vi "rsscope_core_global.vi"() -> ()   [LabVIEW 2014] (continued)
"Descriptive Name"="Advanced Jitter Gating Coupled Zoom Diagram", "Data Type"=6, "Command"="ADVJ{AdvJitterMeas}:SIGN:GATE:ZDI", "Access"=2, "Range Table"="", "Read Callback"="", "Write Callback"="", "Supported Models"="", "Instrument Options"="K133|K134", "Flags"=0, "Help"="Sets the zoom the gate is coupled to, if RSSCOPE_ATTR_ADVANCED_JITTER_GATING_COUPLING_MODE is set to ZOOM.\n\nAvailable Repeated Capabilities:\nAdvJitterMeas: JA1, JA2\r\n\nRemote-control command(s):\nADVJitter<m>:SIGNal:GATE:ZDIagram"}, {"Level"=5, "Class Only"=FALSE, "Identifier"="RSSCOPE_ATTR_ADVANCED_JITTER_GATING_MODE", "Descriptive Name"="Advanced Jitter Gating Mode", "Data Type"=0, "Command"="ADVJ{AdvJitterMeas}:SIGN:GATE:RANG:MODE", "Access"=2, "Range Table"="rsscope_rngAbsRel", "Read Callback"="", "Write Callback"="", "Supported Models"="", "Instrument Options"="K133|K134", "Flags"=0, "Help"="Selects if the gate area is defined in relative values (percent) or absolute.\n\nAvailable Repeated Capabilities:\nAdvJitterMeas: JA1, JA2\r\n\nRemote-control command(s):\nADVJitter<m>:SIGNal:GATE:RANGe:MODE"}, {"Level"=5, "Class Only"=FALSE, "Identifier"="RSSCOPE_ATTR_ADVANCED_JITTER_GATING_ABSOLUTE_START", "Descriptive Name"="Advanced Jitter Gating Absolute Start", "Data Type"=1, "Command"="ADVJ{AdvJitterMeas}:SIGN:GATE:RANG:ABS:STAR", "Access"=2, "Range Table"="RsScope_rngAdvancedJitterGatingRange", "Read Callback"="", "Write Callback"="", "Supported Models"="", "Instrument Options"="K133|K134", "Flags"=0, "Help"="Sets the start time of the gate area in percent, if RSSCOPE_ATTR_ADVANCED_JITTER_GATING_MODE is set to ABS.\n\nAvailable Repeated Capabilities:\nAdvJitterMeas: JA1, JA2\r\n\nRemote-control command(s):\nADVJitter<m>:SIGNal:GATE:RANGe:ABSolute:STARt"}, {"Level"=5, "Class Only"=FALSE, "Identifier"="RSSCOPE_ATTR_ADVANCED_JITTER_GATING_ABSOLUTE_STOP", "Descriptive Name"="Advanced Jitter Gating Absolute Stop", "Data Type"=1, "Command"="ADVJ{AdvJitterMeas}:SIGN:GATE:RANG:ABS:STOP", "Access"=2, "Range Table"="RsScope_rngAdvancedJitterGatingRange", "Read Callback"="", "Write Callback"="", "Supported Models"="", "Instrument Options"="K133|K134", "Flags"=0, "Help"="Sets the stop time of the gate area in percent, if RSSCOPE_ATTR_ADVANCED_JITTER_GATING_MODE is set to ABS.\n\nAvailable Repeated Capabilities:\nAdvJitterMeas: JA1, JA2\r\n\nRemote-control command(s):\nADVJitter<m>:SIGNal:GATE:RANGe:ABSolute:STOP"}, {"Level"=5, "Class Only"=FALSE, "Identifier"="RSSCOPE_ATTR_ADVANCED_JITTER_GATING_RELATIVE_START", "Descriptive Name"="Advanced Jitter Gating Relative Start", "Data Type"=1, "Command"="ADVJ{AdvJitterMeas}:SIGN:GATE:RANG:REL:STAR", "Access"=2, "Range Table"="RsScope_rngPercent", "Read Callback"="", "Write Callback"="", "Supported Models"="", "Instrument Options"="K133|K134", "Flags"=0, "Help"="Sets the relative start of the gate area in percent, if RSSCOPE_ATTR_ADVANCED_JITTER_GATING_MODE is set to REL.\n\nAvailable Repeated Capabilities:\nAdvJitterMeas: JA1, JA2\r\n\nRemote-control command(s):\nADVJitter<m>:SIGNal:GATE:RANGe:RELative:STARt"}, {"Level"=5, "Class Only"=FALSE, "Identifier"="RSSCOPE_ATTR_ADVANCED_JITTER_GATING_RELATIVE_STOP", "Descriptive Name"="Advanced Jitter Gating Relative Stop", "Data Type"=1, "Command"="ADVJ{AdvJitterMeas}:SIGN:GATE:RANG:REL:STOP", "Access"=2, "Range Table"="RsScope_rngPercent", "Read Callback"="", "Write Callback"="", "Supported Models"="", "Instrument Options"="K133|K134", "Flags"=0, "Help"="Sets the relative stop of the gate area in percent, if RSSCOPE_ATTR_ADVANCED_JITTER_GATING_MODE is set to REL.\n\nAvailable Repeated Capabilities:\nAdvJitterMeas: JA1, JA2\r\n\nRemote-control command(s):\nADVJitter<m>:SIGNal:GATE:RANGe:RELative:STOP"}, {"Level"=4, "Class Only"=TRUE, "Identifier"="", "Descriptive Name"="Decomposition", "Data Type"=0, "Command"="", "Access"=0, "Range Table"="", "Read Callback"="", "Write Callback"="", "Supported Models"="", "Instrument Options"="", "Flags"=0, "Help"="This class contains attributes and methods to set the step response of the system and select the jitter components measurements that you want to perform in the advanced jitter measurement subsystem (option K133)"}, {"Level"=5, "Class Only"=FALSE, "Identifier"="RSSCOPE_ATTR_ADVANCED_JITTER_DECOMPOSITION_STEP_RESPONSE_LENGTH", "Descriptive Name"="Advanced Jitter Decomposition Step Response Length", "Data Type"=1, "Command"="ADVJ{AdvJitterMeas}:DCOM:RESP", "Access"=2, "Range Table"="RsScope_rngAdvancedJitterStepResponse", "Read Callback"="", "Write Callback"="", "Supported Models"="", "Instrument Options"="K133|K134", "Flags"=0, "Help"="Set the  step response length in unit intervals.\n\nAvailable Repeated Capabilities:\nAdvJitterMeas: JA1, JA2\r\n\nRemote-control command(s):\nADVJitter<m>:DCOMposition:RESPlength"}, {"Level"=5, "Class Only"=FALSE, "Identifier"="RSSCOPE_ATTR_ADVANCED_JITTER_DECOMPOSITION_ESTIMATE_STEP_RESPONSE", "Descriptive Name"="Advanced Jitter Decomposition Estimate Step Response", "Data Type"=4, "Command"="ADVJ{AdvJitterMeas}:DCOM:RLES", "Access"=1, "Range Table"="", "Read Callback"="", "Write Callback"="", "Supported Models"="", "Instrument Options"="K133|K134", "Flags"=1, "Help"="Estimates the maximum of the reasonable step response length depending on the analyzed signal that guarantees the calculation of the step responses. Tor this, however, a smaller value is also possible, which can be set user-defined with RSSCOPE_ATTR_ADVANCED_JITTER_DECOMPOSITION_STEP_RESPONSE_LENGTH. The user-defined value is overwritten if the estimated maximum is less than the value set by the user.\n\nAvailable Repeated Capabilities:\nAdvJitterMeas: JA1, JA2\r\n\nRemote-control command(s):\nADVJitter<m>:DCOMposition:RLEStimate"}, {"Level"=5, "Class Only"=FALSE, "Identifier"="RSSCOPE_ATTR_ADVANCED_JITTER_DECOMPOSITION_STEP_RESPONSE_ESTIMATED_MAX", "Descriptive Name"="Advanced Jitter Decomposition Step Response Estimated Max", "Data Type"=1, "Command"="ADVJ{AdvJitterMeas}:DCOM:MRES?", "Access"=0, "Range Table"="RsScope_rngAdvancedJitterStepResponse", "Read Callback"="", "Write Callback"="", "Supported Models"="", "Instrument Options"="K133|K134", "Flags"=0, "Help"="Queries the estimated maximum step length response.\n\nAvailable Repeated Capabilities:\nAdvJitterMeas: JA1, JA2\r\n\nRemote-control command(s):\nADVJitter<m>:DCOMposition:MRESplength?"}, {"Level"=5, "Class Only"=FALSE, "Identifier"="RSSCOPE_ATTR_ADVANCED_JITTER_DECOMPOSITION_STEP_POSITION", "Descriptive Name"="Advanced Jitter Decomposition Step Position", "Data Type"=0, "Command"="ADVJ{AdvJitterMeas}:DCOM:POSS", "Access"=2, "Range Table"="rsscope_rngPct", "Read Callback"="", "Write Callback"="", "Supported Models"="", "Instrument Options"="K133|K134", "Flags"=0, "Help"="Sets the steps position. It defines what percentage of the unit lengths are displayed before the step response.\n\nFor example, if the Length is set to 20 UI and the Step position is set to 75%, the step response diagram displays 15 UI before the step response and 5 UI after that.\n\nAvailable Repeated Capabilities:\nAdvJitterMeas: JA1, JA2\r\n\nRemote-control command(s):\nADVJitter<m>:DCOMposition:POSStep"}, {"Level"=5, "Class Only"=FALSE, "Identifier"="RSSCOPE_ATTR_ADVANCED_JITTER_DECOMPOSITION_TARGET_BER_EXPONENT", "Descriptive Name"="Advanced Jitter Decomposition Target BER Exponent", "Data Type"=0, "Command"="ADVJ{AdvJitterMeas}:DCOM:TARB", "Access"=2, "Range Table"="RsScope_rngAdvancedJitterTargetBERExponent", "Read Callback"="", "Write Callback"="", "Supported Models"="", "Instrument Options"="K133|K134", "Flags"=0, "Help"="Sets the target bit error rate for total jitter at BER components. This value is the exponent n where BER = 10^-n.\n\nAvailable Repeated Capabilities:\nAdvJitterMeas: JA1, JA2\r\n\nRemote-control command(s):\nADVJitter<m>:DCOMposition:TARBer"}, {"Level"=5, "Class Only"=FALSE, "Identifier"="RSSCOPE_ATTR_ADVANCED_JITTER_DECOMPOSITION_DISPLAY_INTERLEAVED", "Descriptive Name"="Advanced Jitter Decomposition Display Interleaved", "Data Type"=3, "Command"="ADVJ{AdvJitterMeas}:DCOM:JINT", "Access"=2, "Range Table"="", "Read Callback"="", "Write Callback"="", "Supported Models"="", "Instrument Options"="K133|K134", "Flags"=0, "Help"="Displays interleaved histogram values.\n\nAvailable Repeated Capabilities:\nAdvJitterMeas: JA1, JA2\r\n\nRemote-control command(s):\nADVJitter<m>:DCOMposition:JINTerleaved"}, {"Level"=5, "Class Only"=FALSE, "Identifier"="RSSCOPE_ATTR_ADVANCED_JITTER_DECOMPOSITION_DISPLAY_PERIODIC_JITTER_LABELS", "Descriptive Name"="Advanced Jitter Decomposition Display Periodic Jitter Labels", "Data Type"=3, "Command"="ADVJ{AdvJitterMeas}:DCOM:SPJL", "Access"=2, "Range Table"="", "Read Callback"="", "Write Callback"="", "Supported Models"="", "Instrument Options"="K133|K134", "Flags"=0, "Help"="Enables the display of the periodic jitter components labels.\n\nAvailable Repeated Capabilities:\nAdvJitterMeas: JA1, JA2\r\n\nRemote-control command(s):\nADVJitter<m>:DCOMposition:SPJLabels"}, {"Level"=5, "Class Only"=FALSE, "Identifier"="RSSCOPE_ATTR_ADVANCED_JITTER_DECOMPOSITION_DISPLAY_PERIODIC_NOISE_LABELS", "Descriptive Name"="Advanced Jitter Decomposition Display Periodic Noise Labels", "Data Type"=3, "Command"="ADVJ{AdvJitterMeas}:DCOM:SPNL", "Access"=2, "Range Table"="", "Read Callback"="", "Write Callback"="", "Supported Models"="", "Instrument Options"="K133|K134", "Flags"=0, "Help"="Enables the display of the periodic noise components labels.\n\nAvailable Repeated Capabilities:\nAdvJitterMeas: JA1, JA2\r\n\nRemote-control command(s):\nADVJitter<m>:DCOMposition:SPNLabels"}, {"Level"=5, "Class Only"=TRUE, "Identifier"="", "Descriptive Name"="Components", "Data Type"=0, "Command"="", "Access"=0, "Range Table"="", "Read Callback"="", "Write Callback"="", "Supported Models"="", "Instrument Options"="", "Flags"=0, "Help"="This class contains methods that enable and configure jitter decomposition components in the advanced jitter measurement subsystem (option K133)"}, {"Level"=6, "Class Only"=FALSE, "Identifier"="RSSCOPE_ATTR_ADVANCED_JITTER_DECOMPOSITION_SELECT_ALL_BASIC_JITTER_COMPONENTS", "Descriptive Name"="Advanced Jitter Decomposition Select All Basic Jitter Components", "Data Type"=4, "Command"="ADVJ{AdvJitterMeas}:DCOM:SELB", "Access"=1, "Range Table"="", "Read Callback"="", "Write Callback"="", "Supported Models"="", "Instrument Options"="K133|K134", "Flags"=0, "Help"="Selects all basic jitter components.\n\nAvailable Repeated Capabilities:\nAdvJitterMeas: JA1, JA2\r\n\nRemote-control command(s):\nADVJitter<m>:DCOMposition:SELBasicmeas"}, {"Level"=6, "Class Only"=FALSE, "Identifier"="RSSCOPE_ATTR_ADVANCED_JITTER_DECOMPOSITION_SELECT_ALL_JITTER_COMPONENTS", "Descriptive Name"="Advanced Jitter Decomposition Select All Jitter Components", "Data Type"=4, "Command"="ADVJ{AdvJitterMeas}:DCOM:SELJ", "Access"=1, "Range Table"="", "Read Callback"="", "Write Callback"="", "Supported Models"="", "Instrument Options"="K133|K134", "Flags"=0, "Help"="Selects all jitter components.\n\nAvailable Repeated Capabilities:\nAdvJitterMeas: JA1, JA2\r\n\nRemote-control command(s):\nADVJitter<m>:DCOMposition:SELJitcomp"}, {"Level"=6, "Class Only"=FALSE, "Identifier"="RSSCOPE_ATTR_ADVANCED_JITTER_DECOMPOSITION_CLEAR_SELECTED_BASIC_JITTER_COMPONENTS", "Descriptive Name"="Advanced Jitter Decomposition Clear Selected Basic Jitter Components", "Data Type"=4, "Command"="ADVJ{AdvJitterMeas}:DCOM:CLEB", "Access"=1, "Range Table"="", "Read Callback"="", "Write Callback"="", "Supported Models"="", "Instrument Options"="K133|K134", "Flags"=0, "Help"="Clears all selected basic jitter components.\n\nAvailable Repeated Capabilities:\nAdvJitterMeas: JA1, JA2\r\n\nRemote-control command(s):\nADVJitter<m>:DCOMposition:CLEBasicmeas"}, {"Level"=6, "Class Only"=FALSE, "Identifier"="RSSCOPE_ATTR_ADVANCED_JITTER_DECOMPOSITION_CLEAR_SELECTED_JITTER_COMPONENTS", "Descriptive Name"="Advanced Jitter Decomposition Clear Selected Jitter Components", "Data Type"=4, "Command"="ADVJ{AdvJitterMeas}:DCOM:CLEJ", "Access"=1, "Range Table"="", "Read Callback"="", "Write Callback"="", "Supported Models"="", "Instrument Options"="K133|K134", "Flags"=0, "Help"="Clears all selected jitter components.\n\nAvailable Repeated Capabilities:\nAdvJitterMeas: JA1, JA2\r\n\nRemote-control command(s):\nADVJitter<m>:DCOMposition:CLEJitcomp"}, {"Level"=6, "Class Only"=FALSE, "Identifier"="RSSCOPE_ATTR_ADVANCED_JITTER_DECOMPOSITION_COMPONENT_ENABLED", "Descriptive Name"="Advanced Jitter Decomposition Component Enabled", "Data Type"=3, "Command"="ADVJ{AdvJitterMeas}:DCOM:COMP{AdvJitterComponent}:ENAB", "Access"=2, "Range Table"="", "Read Callback"="", "Write Callback"="", "Supported Models"="", "Instrument Options"="K133|K134", "Flags"=0, "Help"="Enables the measurement for the specified jitter component.\n\nAvailable Repeated Capabilities:\nAdvJitterMeas: JA1, JA2\r\nAdvJitterComponent: f_symb, T_symb, EC, TJ_BER, RJ, DDirac, TJ, DJ, DDJ, DCD, PJ, ISI\r\n\nRemote-control command(s):\nADVJitter<m>:DCOMposition:COMPonents<n>:ENABle"}, {"Level"=6, "Class Only"=FALSE, "Identifier"="RSSCOPE_ATTR_ADVANCED_JITTER_DECOMPOSITION_SELECT_ALL_NOISE_COMPONENTS", "Descriptive Name"="Advanced Jitter Decomposition Select All Noise Components", "Data Type"=4, "Command"="ADVJ{AdvJitterMeas}:DCOM:SELN", "Access"=1, "Range Table"="", "Read Callback"="", "Write Callback"="", "Supported Models"="", "Instrument Options"="K133|K134", "Flags"=0, "Help"="Selects all noise components.\n\nAvailable Repeated Capabilities:\nAdvJitterMeas: JA1, JA2\r\n\nRemote-control command(s):\nADVJitter<m>:DCOMposition:SELNoisecomp"}, {"Level"=6, "Class Only"=FALSE, "Identifier"="RSSCOPE_ATTR_ADVANCED_JITTER_DECOMPOSITION_CLEAR_SELECTED_NOISE_COMPONENTS", "Descriptive Name"="Advanced Jitter Decomposition Clear Selected Noise Components", "Data Type"=4, "Command"="ADVJ{AdvJitterMeas}:DCOM:CLEN", "Access"=1, "Range Table"="", "Read Callback"="", "Write Callback"="", "Supported Models"="", "Instrument Options"="K133|K134", "Flags"=0, "Help"="Clears all selected noise components.\n\nAvailable Repeated Capabilities:\nAdvJitterMeas: JA1, JA2\r\n\nRemote-control command(s):\nADVJitter<m>:DCOMposition:CLENoisecomp"}, {"Level"=6, "Class Only"=FALSE, "Identifier"="RSSCOPE_ATTR_ADVANCED_JITTER_DECOMPOSITION_PERIODIC_COMPONENTS_ENABLED", "Descriptive Name"="Advanced Jitter Decomposition Periodic Components Enabled", "Data Type"=3, "Command"="ADVJ{AdvJitterMeas}:DCOM:ENP", "Access"=2, "Range Table"="", "Read Callback"="", "Write Callback"="", "Supported Models"="", "Instrument Options"="K133|K134", "Flags"=0, "Help"="Enables the display of the periodic jitter components table.\n\nAvailable Repeated Capabilities:\nAdvJitterMeas: JA1, JA2\r\n\nRemote-control command(s):\nADVJitter<m>:DCOMposition:ENP"}, {"Level"=6, "Class Only"=FALSE, "Identifier"="RSSCOPE_ATTR_ADVANCED_JITTER_DECOMPOSITION_MAX_PERIODIC_VERTICAL_COMPONENTS", "Descriptive Name"="Advanced Jitter Decomposition Max Periodic Vertical Components", "Data Type"=0, "Command"="ADVJ{AdvJitterMeas}:DCOM:NVER", "Access"=2, "Range Table"="RsScope_rngAdvancedJitterPeriodicComponents", "Read Callback"="", "Write Callback"="", "Supported Models"="", "Instrument Options"="K133|K134", "Flags"=0, "Help"="Sets the maximum number of periodic components in the vertical direction that are considered for the measurement. If the actual number of periodic components is higher than the set value, they are considered for the random jitter component.\n\nAvailable Repeated Capabilities:\nAdvJitterMeas: JA1, JA2\r\n\nRemote-control command(s):\nADVJitter<m>:DCOMposition:NVERtical"}, {"Level"=6, "Class Only"=FALSE, "Identifier"="RSSCOPE_ATTR_ADVANCED_JITTER_DECOMPOSITION_MAX_PERIODIC_HORIZONTAL_COMPONENTS", "Descriptive Name"="Advanced Jitter Decomposition Max Periodic Horizontal Components", "Data Type"=0, "Command"="ADVJ{AdvJitterMeas}:DCOM:NHOR", "Access"=2, "Range Table"="RsScope_rngAdvancedJitterPeriodicComponents", "Read Callback"="", "Write Callback"="", "Supported Models"="", "Instrument Options"="K133|K134", "Flags"=0, "Help"="Sets the maximum number of periodic components in the horizontal direction that are considered for the measurement. If the actual number of periodic components is higher than the set value, they are considered for the random jitter component.\n\nAvailable Repeated Capabilities:\nAdvJitterMeas: JA1, JA2\r\n\nRemote-control command(s):\nADVJitter<m>:DCOMposition:NHORizontal"}, {"Level"=6, "Class Only"=FALSE, "Identifier"="RSSCOPE_ATTR_ADVANCED_JITTER_DECOMPOSITION_OTHER_BOUNDED_UNCORRELATED_ENABLED", "Descriptive Name"="Advanced Jitter Decomposition Other Bounded Uncorrelated Enabled", "Data Type"=3, "Command"="ADVJ{AdvJitterMeas}:DCOM:ENOB", "Access"=2, "Range Table"="", "Read Callback"="", "Write Callback"="", "Supported Models"="", "Instrument Options"="K133|K134", "Flags"=0, "Help"="If enabled, allows the selection of the (other) bounded uncorrelated jitter/noise: (O)BUJ, (O)BUJ(d -d) , RJ, (O)BUN, (O)BUN(d -d) , RN.\n\nThe other bounded uncorrelated jitter/noise includes the periodic jitter/noise components. It is displayed, if Periodic is enabled. Otherwise the bounded uncorrelated jitter/noise is displayed.\n\nAvailable Repeated Capabilities:\nAdvJitterMeas: JA1, JA2\r\n\nRemote-control command(s):\nADVJitter<m>:DCOMposition:ENOBu"}, {"Level"=6, "Class Only"=FALSE, "Identifier"="RSSCOPE_ATTR_ADVANCED_JITTER_DECOMPOSITION_PERIODIC_JITTER_TABLE_ENABLED", "Descriptive Name"="Advanced Jitter Decomposition Periodic Jitter Table Enabled", "Data Type"=3, "Command"="ADVJ{AdvJitterMeas}:DCOM:SPJT", "Access"=2, "Range Table"="", "Read Callback"="", "Write Callback"="", "Supported Models"="", "Instrument Options"="K133|K134", "Flags"=0, "Help"="Enables the display of the periodic jitter components table.\n\nAvailable Repeated Capabilities:\nAdvJitterMeas: JA1, JA2\r\n\nRemote-control command(s):\nADVJitter<m>:DCOMposition:SPJTable"}, {"Level"=4, "Class Only"=TRUE, "Identifier"="", "Descriptive Name"="Results", "Data Type"=0, "Command"="", "Access"=0, "Range Table"="", "Read Callback"="", "Write Callback"="", "Supported Models"="", "Instrument Options"="", "Flags"=0, "Help"="This class provides access to your measurement results in the advanced jitter measurement subsystem (option K133)"}, {"Level"=5, "Class Only"=FALSE, "Identifier"="RSSCOPE_ATTR_ADVANCED_JITTER_RESULTS_ENABLED", "Descriptive Name"="Advanced Jitter Results Enabled", "Data Type"=3, "Command"="ADVJ{AdvJitterMeas}:RES:ENAB", "Access"=2, "Range Table"="", "Read Callback"="", "Write Callback"="", "Supported Models"="", "Instrument Options"="K133|K134", "Flags"=0, "Help"="Enables the advanced jitter analysis. It displays all enabled diagrams and displays a table with the results for the component measurements.\n\nAvailable Repeated Capabilities:\nAdvJitterMeas: JA1, JA2\r\n\nRemote-control command(s):\nADVJitter<m>:RESult:ENABle"}, {"Level"=5, "Class Only"=FALSE, "Identifier"="RSSCOPE_ATTR_ADVANCED_JITTER_RESULTS_STATISTICS_ENABLED", "Descriptive Name"="Advanced Jitter Results Statistics Enabled", "Data Type"=3, "Command"="ADVJ{AdvJitterMeas}:RES:STAT", "Access"=2, "Range Table"="", "Read Callback"="", "Write Callback"="", "Supported Models"="", "Instrument Options"="K133|K134", "Flags"=0, "Help"="Enables statistics measurements for the advanced jitter analysis.\n\nAvailable Repeated Capabilities:\nAdvJitterMeas: JA1, JA2\r\n\nRemote-control command(s):\nADVJitter<m>:RESult:STATistics"}, {"Level"=5, "Class Only"=FALSE, "Identifier"="RSSCOPE_ATTR_ADVANCED_JITTER_RESULTS_STEP_RESPONSE_DIAGRAM_ENABLED", "Descriptive Name"="Advanced Jitter Results Step Response Diagram Enabled", "Data Type"=3, "Command"="ADVJ{AdvJitterMeas}:RES:STEP", "Access"=2, "Range Table"="", "Read Callback"="", "Write Callback"="", "Supported Models"="", "Instrument Options"="K133|K134", "Flags"=0, "Help"="Enables a step response diagram for the advanced jitter measurements.\n\nAvailable Repeated Capabilities:\nAdvJitterMeas: JA1, JA2\r\n\nRemote-control command(s):\nADVJitter<m>:RESult:STEPresponse"}, {"Level"=5, "Class Only"=FALSE, "Identifier"="RSSCOPE_ATTR_ADVANCED_JITTER_RESULTS_BATHTUB_PLOT_ENABLED", "Descriptive Name"="Advanced Jitter Results Bathtub Plot Enabled", "Data Type"=3, "Command"="ADVJ{AdvJitterMeas}:RES:BATH", "Access"=2, "Range Table"="", "Read Callback"="", "Write Callback"="", "Supported Models"="", "Instrument Options"="K133|K134", "Flags"=0, "Help"="Enables a bathtub plot for the advanced jitter measurements.\n\nAvailable Repeated Capabilities:\nAdvJitterMeas: JA1, JA2\r\n\nRemote-control command(s):\nADVJitter<m>:RESult:BATHtub"}, {"Level"=5, "Class Only"=FALSE, "Identifier"="RSSCOPE_ATTR_ADVANCED_JITTER_RESULTS_BATHTUB_PLOT_TYPE", "Descriptive Name"="Advanced Jitter Results Bathtub Plot Type", "Data Type"=0, "Command"="ADVJ{AdvJitterMeas}:RES:TYPB", "Access"=2, "Range Table"="RsScope_rngAdvancedJitterResultsBathtubPlotType", "Read Callback"="", "Write Callback"="", "Supported Models"="", "Instrument Options"="K133|K134", "Flags"=0, "Help"="Selects if you want to display the bathtub results versus total jitter (TJ) or data-dependent jitter (DDJ) and random jitter (RJ) components.\n\nAvailable Repeated Capabilities:\nAdvJitterMeas: JA1, JA2\r\n\nRemote-control command(s):\nADVJitter<m>:RESult:TYPBathtub"}, {"Level"=5, "Class Only"=FALSE, "Identifier"="RSSCOPE_ATTR_ADVANCED_JITTER_RESULTS_BATHTUB_PERIODIC_COMPONENTS_ENABLED", "Descriptive Name"="Advanced Jitter Results Bathtub Periodic Components Enabled", "Data Type"=3, "Command"="ADVJ{AdvJitterMeas}:RES:PJ", "Access"=2, "Range Table"="", "Read Callback"="", "Write Callback"="", "Supported Models"="", "Instrument Options"="K133|K134", "Flags"=0, "Help"="If enabled, the periodic jitter components are considered for the jitter bathtub. Requires periodic components to be enabled (RSSCOPE_ATTR_ADVANCED_JITTER_DECOMPOSITION_PERIODIC_COMPONENTS_ENABLED).\n\nAvailable Repeated Capabilities:\nAdvJitterMeas: JA1, JA2\r\n\nRemote-control command(s):\nADVJitter<m>:RESult:PJ"}, {"Level"=5, "Class Only"=FALSE, "Identifier"="RSSCOPE_ATTR_ADVANCED_JITTER_RESULTS_BATHTUB_OBUJ_COMPONENTS_ENABLED", "Descriptive Name"="Advanced Jitter Results Bathtub OBUJ Components Enabled", "Data Type"=3, "Command"="ADVJ{AdvJitterMeas}:RES:OBUJ", "Access"=2, "Range Table"="", "Read Callback"="", "Write Callback"="", "Supported Models"="", "Instrument Options"="K133|K134", "Flags"=0, "Help"="If enabled, the other bounded uncorrelated jitter components are considered for the jitter bathtub. Requires other bounded uncorrelated components to be enabled (RSSCOPE_ATTR_ADVANCED_JITTER_DECOMPOSITION_OTHER_BOUNDED_UNCORRELATED_ENABLED).\n\nAvailable Repeated Capabilities:\nAdvJitterMeas: JA1, JA2\r\n\nRemote-control command(s):\nADVJitter<m>:RESult:OBUJ"}, {"Level"=5, "Class Only"=FALSE, "Identifier"="RSSCOPE_ATTR_ADVANCED_JITTER_RESULTS_NOISE_BATHTUB_PLOT_ENABLED", "Descriptive Name"="Advanced Jitter Results Noise Bathtub Plot Enabled", "Data Type"=3, "Command"="ADVJ{AdvJitterMeas}:RES:NBAT", "Access"=2, "Range Table"="", "Read Callback"="", "Write Callback"="", "Supported Models"="", "Instrument Options"="K133|K134", "Flags"=0, "Help"="Enables a noise bathtub plot, a graph of BER in a log scale versus data-dependent jitter (DDN).\n\nAvailable Repeated Capabilities:\nAdvJitterMeas: JA1, JA2\r\n\nRemote-control command(s):\nADVJitter<m>:RESult:NBAThtub"}, {"Level"=5, "Class Only"=FALSE, "Identifier"="RSSCOPE_ATTR_ADVANCED_JITTER_RESULTS_NOISE_BATHTUB_PERIODIC_COMPONENTS_ENABLED", "Descriptive Name"="Advanced Jitter Results Noise Bathtub Periodic Components Enabled", "Data Type"=3, "Command"="ADVJ{AdvJitterMeas}:RES:PN", "Access"=2, "Range Table"="", "Read Callback"="", "Write Callback"="", "Supported Models"="", "Instrument Options"="K133|K134", "Flags"=0, "Help"="If enabled, the periodic noise components are considered for the noise bathtub. Requires periodic components to be enabled (RSSCOPE_ATTR_ADVANCED_JITTER_DECOMPOSITION_PERIODIC_COMPONENTS_ENABLED).\n\nAvailable Repeated Capabilities:\nAdvJitterMeas: JA1, JA2\r\n\nRemote-control command(s):\nADVJitter<m>:RESult:PN"}, {"Level"=5, "Class Only"=FALSE, "Identifier"="RSSCOPE_ATTR_ADVANCED_JITTER_RESULTS_NOISE_BATHTUB_OBUN_COMPONENTS_ENABLED", "Descriptive Name"="Advanced Jitter Results Noise Bathtub OBUN Components Enabled", "Data Type"=3, "Command"="ADVJ{AdvJitterMeas}:RES:OBUN", "Access"=2, "Range Table"="", "Read Callback"="", "Write Callback"="", "Supported Models"="", "Instrument Options"="K133|K134", "Flags"=0, "Help"="If enabled, the other bounded uncorrelated noise components are considered for the noise bathtub. Requires other bounded uncorrelated components to be enabled (RSSCOPE_ATTR_ADVANCED_JITTER_DECOMPOSITION_OTHER_BOUNDED_UNCORRELATED_ENABLED).\n\nAvailable Repeated Capabilities:\nAdvJitterMeas: JA1, JA2\r\n\nRemote-control command(s):\nADVJitter<m>:RESult:OBUN"}, {"Level"=5, "Class Only"=FALSE, "Identifier"="RSSCOPE_ATTR_ADVANCED_JITTER_RESULTS_SYNTHETIC_EYE_PLOT_ENABLED", "Descriptive Name"="Advanced Jitter Results Synthetic Eye Plot Enabled", "Data Type"=3, "Command"="ADVJ{AdvJitterMeas}:RES:SYNT", "Access"=2, "Range Table"="", "Read Callback"="", "Write Callback"="", "Supported Models"="", "Instrument Options"="K133|K134", "Flags"=0, "Help"="Selects if you want to display synthetic eye results only for the deterministic jitter (DJ) components or the data-dependent jitter (DDJ) components.\n\nAvailable Repeated Capabilities:\nAdvJitterMeas: JA1, JA2\r\n\nRemote-control command(s):\nADVJitter<m>:RESult:SYNTheticeye"}, {"Level"=5, "Class Only"=FALSE, "Identifier"="RSSCOPE_ATTR_ADVANCED_JITTER_RESULTS_SYNTHETIC_EYE_PLOT_TYPE", "Descriptive Name"="Advanced Jitter Results Synthetic Eye Plot Type", "Data Type"=0, "Command"="ADVJ{AdvJitterMeas}:RES:TYPS", "Access"=2, "Range Table"="RsScope_rngAdvancedJitterSyntheticEyePlot", "Read Callback"="", "Write Callback"="", "Supported Models"="", "Instrument Options"="K133|K134", "Flags"=0, "Help"="Selects if you want to display synthetic eye results only for the deterministic jitter (DDP) components or the data-dependent jitter (DD) components.\n\nAvailable Repeated Capabilities:\nAdvJitterMeas: JA1, JA2\r\n\nRemote-control command(s):\nADVJitter<m>:RESult:TYPSynteye"}, {"Level"=5, "Class Only"=FALSE, "Identifier"="RSSCOPE_ATTR_ADVANCED_JITTER_RESULTS_SYNTHETIC_EYE_HORIZONTAL_COMPONENTS_ENABLED", "Descriptive Name"="Advanced Jitter Results Synthetic Eye Horizontal Components Enabled", "Data Type"=3, "Command"="ADVJ{AdvJitterMeas}:RES:PHOR", "Access"=2, "Range Table"="", "Read Callback"="", "Write Callback"="", "Supported Models"="", "Instrument Options"="K133|K134", "Flags"=0, "Help"="If enabled, adds horizontal periodic components to the data-dependent synthetic eye.\n\nAvailable Repeated Capabilities:\nAdvJitterMeas: JA1, JA2\r\n\nRemote-control command(s):\nADVJitter<m>:RESult:PHORizontal"}, {"Level"=5, "Class Only"=FALSE, "Identifier"="RSSCOPE_ATTR_ADVANCED_JITTER_RESULTS_SYNTHETIC_EYE_VERTICAL_COMPONENTS_ENABLED", "Descriptive Name"="Advanced Jitter Results Synthetic Eye Vertical Components Enabled", "Data Type"=3, "Command"="ADVJ{AdvJitterMeas}:RES:PVER", "Access"=2, "Range Table"="", "Read Callback"="", "Write Callback"="", "Supported Models"="", "Instrument Options"="K133|K134", "Flags"=0, "Help"="If enabled, adds vertical periodic components to the data-dependent synthetic eye.\n\nAvailable Repeated Capabilities:\nAdvJitterMeas: JA1, JA2\r\n\nRemote-control command(s):\nADVJitter<m>:RESult:PVERtical"}, {"Level"=5, "Class Only"=FALSE, "Identifier"="RSSCOPE_ATTR_ADVANCED_JITTER_RESULTS_DIAGRAM_TRANSITIONS", "Descriptive Name"="Advanced Jitter Results Diagram Transitions", "Data Type"=0, "Command"="ADVJ{AdvJitterMeas}:RES:TRAN", "Access"=2, "Range Table"="RsScope_rngAdvancedJitterResultsDiagramTransitions", "Read Callback"="", "Write Callback"="", "Supported Models"="", "Instrument Options"="K133|K134", "Flags"=0, "Help"="Selects which transitions are considered for the display of the diagrams, rising, falling or both. This setting is mostly relevant for histograms, tracks and the measurement results.\n\nAvailable Repeated Capabilities:\nAdvJitterMeas: JA1, JA2\r\n\nRemote-control command(s):\nADVJitter<m>:RESult:TRANsitions"}, {"Level"=5, "Class Only"=FALSE, "Identifier"="RSSCOPE_ATTR_ADVANCED_JITTER_RESULTS_DIAGRAM_LEVELS", "Descriptive Name"="Advanced Jitter Results Diagram Levels", "Data Type"=0, "Command"="ADVJ{AdvJitterMeas}:RES:LEV", "Access"=2, "Range Table"="RsScope_rngAdvancedJitterResultsDiagramLevels", "Read Callback"="", "Write Callback"="", "Supported Models"="", "Instrument Options"="K133|K134", "Flags"=0, "Help"="Selects which levels are considered for the display of the diagrams, rising, falling or both. This setting is mostly relevant for histograms, tracks and the measurement results.\n\nAvailable Repeated Capabilities:\nAdvJitterMeas: JA1, JA2\r\n\nRemote-control command(s):\nADVJitter<m>:RESult:LEVels"}, {"Level"=5, "Class Only"=FALSE, "Identifier"="RSSCOPE_ATTR_ADVANCED_JITTER_RESULTS_UNIT", "Descriptive Name"="Advanced Jitter Results Unit", "Data Type"=0, "Command"="ADVJ{AdvJitterMeas}:RES:UNIT", "Access"=2, "Range Table"="rsscope_rngAbsRel", "Read Callback"="", "Write Callback"="", "Supported Models"="", "Instrument Options"="K133|K134", "Flags"=0, "Help"="Selects between the absolute and relative unit for the displayed results.\n\nAvailable Repeated Capabilities:\nAdvJitterMeas: JA1, JA2\r\n\nRemote-control command(s):\nADVJitter<m>:RESult:UNIT"}, {"Level"=5, "Class Only"=TRUE, "Identifier"="", "Descriptive Name"="Component", "Data Type"=0, "Command"="", "Access"=0, "Range Table"="", "Read Callback"="", "Write Callback"="", "Supported Models"="", "Instrument Options"="", "Flags"=0, "Help"="This class contains methods that enable and configure the display of jitter decomposition component results in the advanced jitter measurement subsystem (option K133)"}, {"Level"=6, "Class Only"=FALSE, "Identifier"="RSSCOPE_ATTR_ADVANCED_JITTER_RESULTS_COMPONENT_HISTOGRAM_ENABLED", "Descriptive Name"="Advanced Jitter Results Component Histogram Enabled", "Data Type"=3, "Command"="ADVJ{AdvJitterMeas}:RES:COMP{AdvJitterComponent}:HIST", "Access"=2, "Range Table"="", "Read Callback"="", "Write Callback"="", "Supported Models"="", "Instrument Options"="K133|K134", "Flags"=0, "Help"="Enables a histogram for the selected measurement component. Valid for f_symb, T_symb, RJ, TJ, DJ, DDJ, and PJ components.\n\nAvailable Repeated Capabilities:\nAdvJitterMeas: JA1, JA2\r\nAdvJitterComponent: f_symb, T_symb, EC, TJ_BER, RJ, DDirac, TJ, DJ, DDJ, DCD, PJ, ISI\r\n\nRemote-control command(s):\nADVJitter<m>:RESult:COMPonents<n>:HISTogram"}, {"Level"=6, "Class Only"=FALSE, "Identifier"="RSSCOPE_ATTR_ADVANCED_JITTER_RESULTS_COMPONENT_TRACK_ENABLED", "Descriptive Name"="Advanced Jitter Results Component Track Enabled", "Data Type"=3, "Command"="ADVJ{AdvJitterMeas}:RES:COMP{AdvJitterComponent}:TRAC", "Access"=2, "Range Table"="", "Read Callback"="", "Write Callback"="", "Supported Models"="", "Instrument Options"="K133|K134", "Flags"=0, "Help"="Enables a track for the advanced jitter measurements. Valid for f_symb, T_symb, RJ, TJ, DDJ, and PJ components.\n\nAvailable Repeated Capabilities:\nAdvJitterMeas: JA1, JA2\r\nAdvJitterComponent: f_symb, T_symb, EC, TJ_BER, RJ, DDirac, TJ, DJ, DDJ, DCD, PJ, ISI\r\n\nRemote-control command(s):\nADVJitter<m>:RESult:COMPonents<n>:TRACk"}, {"Level"=6, "Class Only"=FALSE, "Identifier"="RSSCOPE_ATTR_ADVANCED_JITTER_RESULTS_COMPONENT_SPECTRUM_ENABLED", "Descriptive Name"="Advanced Jitter Results Component Spectrum Enabled", "Data Type"=3, "Command"="ADVJ{AdvJitterMeas}:RES:COMP{AdvJitterComponent}:SPEC", "Access"=2, "Range Table"="", "Read Callback"="", "Write Callback"="", "Supported Models"="", "Instrument Options"="K133|K134", "Flags"=0, "Help"="Enables a spectrum diagram for the selected measurement component. Valid for RJ, TJ, DDJ, and PJ components.\n\nAvailable Repeated Capabilities:\nAdvJitterMeas: JA1, JA2\r\nAdvJitterComponent: f_symb, T_symb, EC, TJ_BER, RJ, DDirac, TJ, DJ, DDJ, DCD, PJ, ISI\r\n\nRemote-control command(s):\nADVJitter<m>:RESult:COMPonents<n>:SPECtrum"}, {"Level"=6, "Class Only"=FALSE, "Identifier"="RSSCOPE_ATTR_ADVANCED_JITTER_RESULTS_COMPONENT_SCALE", "Descriptive Name"="Advanced Jitter Results Component Scale", "Data Type"=1, "Command"="ADVJ{AdvJitterMeas}:RES:COMP{AdvJitterComponent}:SCAL", "Access"=2, "Range Table"="RsScope_rngAdvancedJitterResultsScale", "Read Callback"="", "Write Callback"="", "Supported Models"="", "Instrument Options"="K133|K134", "Flags"=0, "Help"="Sets the scale for the selected component. Requires RSSCOPE_ATTR_ADVANCED_JITTER_RESULTS_CONTINUOUS_AUTO_SCALE_ENABLED to be off. Units depend on which value is being set. You can set separate scale values for:\n- Symbol rate (in Baud)\n- Symbol duration (in s/div)\n- One scale value that is relevant for all advanced jitter components (in s/div)\n\nAvailable Repeated Capabilities:\nAdvJitterMeas: JA1, JA2\r\nAdvJitterComponent: f_symb, T_symb, EC, TJ_BER, RJ, DDirac, TJ, DJ, DDJ, DCD, PJ, ISI\r\n\nRemote-control command(s):\nADVJitter<m>:RESult:COMPonents<n>:SCALe"}, {"Level"=6, "Class Only"=FALSE, "Identifier"="RSSCOPE_ATTR_ADVANCED_JITTER_RESULTS_COMPONENT_OFFSET", "Descriptive Name"="Advanced Jitter Results Component Offset", "Data Type"=1, "Command"="ADVJ{AdvJitterMeas}:RES:COMP{AdvJitterComponent}:OFFS", "Access"=2, "Range Table"="RsScope_rngAdvancedJitterResultsOffset", "Read Callback"="", "Write Callback"="", "Supported Models"="", "Instrument Options"="K133|K134", "Flags"=0, "Help"="Sets the offest for the selected component. Requires RSSCOPE_ATTR_ADVANCED_JITTER_RESULTS_CONTINUOUS_AUTO_SCALE_ENABLED to be off. Units depend on which value is being set. You can set separate offset values for:\n- Symbol rate (in Baud)\n- Symbol duration (in s/div)\n- One offset value that is relevant for all advanced jitter components (in s/div)\n\nAvailable Repeated Capabilities:\nAdvJitterMeas: JA1, JA2\r\nAdvJitterComponent: f_symb, T_symb, EC, TJ_BER, RJ, DDirac, TJ, DJ, DDJ, DCD, PJ, ISI\r\n\nRemote-control command(s):\nADVJitter<m>:RESult:COMPonents<n>:OFFSet"}, {"Level"=6, "Class Only"=FALSE, "Identifier"="RSSCOPE_ATTR_ADVANCED_JITTER_RESULTS_COMPONENT_PEAK_TO_PEAK", "Descriptive Name"="Advanced Jitter Results Component Peak To Peak", "Data Type"=1, "Command"="ADVJ{AdvJitterMeas}:RES:COMP{AdvJitterComponent}:PEAK?", "Access"=0, "Range Table"="", "Read Callback"="", "Write Callback"="", "Supported Models"="", "Instrument Options"="K133|K134", "Flags"=0, "Help"="Queries the absolute/peak to peak value of the specified jitter component.\n\nAvailable Repeated Capabilities:\nAdvJitterMeas: JA1, JA2\r\nAdvJitterComponent: f_symb, T_symb, EC, TJ_BER, RJ, DDirac, TJ, DJ, DDJ, DCD, PJ, ISI\r\n\nRemote-control command(s):\nADVJitter<m>:RESult:COMPonents<n>:PEAKpeak?"}, {"Level"=6, "Class Only"=FALSE, "Identifier"="RSSCOPE_ATTR_ADVANCED_JITTER_RESULTS_COMPONENT_STANDARD_DEVIATION", "Descriptive Name"="Advanced Jitter Results Component Standard Deviation", "Data Type"=1, "Command"="ADVJ{AdvJitterMeas}:RES:COMP{AdvJitterComponent}:STDD?", "Access"=0, "Range Table"="", "Read Callback"="", "Write Callback"="", "Supported Models"="", "Instrument Options"="K133|K134", "Flags"=0, "Help"="Queries the standard deviation value of the selected component.\n\nAvailable Repeated Capabilities:\nAdvJitterMeas: JA1, JA2\r\nAdvJitterComponent: f_symb, T_symb, EC, TJ_BER, RJ, DDirac, TJ, DJ, DDJ, DCD, PJ, ISI\r\n\nRemote-control command(s):\nADVJitter<m>:RESult:COMPonents<n>:STDDev?"}, {"Level"=6, "Class Only"=FALSE, "Identifier"="RSSCOPE_ATTR_ADVANCED_JITTER_RESULTS_COMPONENT_STATISTICS_WAVEFORM_COUNT", "Descriptive Name"="Advanced Jitter Results Component Statistics Waveform Count", "Data Type"=5, "Command"="ADVJ{AdvJitterMeas}:RES:COMP{AdvJitterComponent}:STAT:WFMC?", "Access"=0, "Range Table"="", "Read Callback"="", "Write Callback"="", "Supported Models"="", "Instrument Options"="K133|K134", "Flags"=0, "Help"="Returns the number of waveforms (acquisitions) the measurement is based on for the specified measurement component.\n\nAvailable Repeated Capabilities:\nAdvJitterMeas: JA1, JA2\r\nAdvJitterComponent: f_symb, T_symb, EC, TJ_BER, RJ, DDirac, TJ, DJ, DDJ, DCD, PJ, ISI\r\n\nRemote-control command(s):\nADVJitter<m>:RESult:COMPonents<n>:STATistics:WFMCount?"}, {"Level"=6, "Class Only"=FALSE, "Identifier"="RSSCOPE_ATTR_ADVANCED_JITTER_RESULTS_COMPONENT_STATISTICS_MAX_PEAK_TO_PEAK", "Descriptive Name"="Advanced Jitter Results Component Statistics Max Peak To Peak", "Data Type"=1, "Command"="ADVJ{AdvJitterMeas}:RES:COMP{AdvJitterComponent}:STAT:MAXP?", "Access"=0, "Range Table"="", "Read Callback"="", "Write Callback"="", "Supported Models"="", "Instrument Options"="K133|K134", "Flags"=0, "Help"="Returns the absolute maximum value of the specified measurement component.\n\nAvailable Repeated Capabilities:\nAdvJitterMeas: JA1, JA2\r\nAdvJitterComponent: f_symb, T_symb, EC, TJ_BER, RJ, DDirac, TJ, DJ, DDJ, DCD, PJ, ISI\r\n\nRemote-control command(s):\nADVJitter<m>:RESult:COMPonents<n>:STATistics:MAXPeakpeak?"}, {"Level"=6, "Class Only"=FALSE, "Identifier"="RSSCOPE_ATTR_ADVANCED_JITTER_RESULTS_COMPONENT_STATISTICS_MAX_STANDARD_DEVIATION", "Descriptive Name"="Advanced Jitter Results Component Statistics Max Standard Deviation", "Data Type"=1, "Command"="ADVJ{AdvJitterMeas}:RES:COMP{AdvJitterComponent}:STAT:MAXS?", "Access"=0, "Range Table"="", "Read Callback"="", "Write Callback"="", "Supported Models"="", "Instrument Options"="K133|K134", "Flags"=0, "Help"="Return the standard deviation of the maximum value of the specified measurement component.\n\nAvailable Repeated Capabilities:\nAdvJitterMeas: JA1, JA2\r\nAdvJitterComponent: f_symb, T_symb, EC, TJ_BER, RJ, DDirac, TJ, DJ, DDJ, DCD, PJ, ISI\r\n\nRemote-control command(s):\nADVJitter<m>:RESult:COMPonents<n>:STATistics:MAXStddev?"}, {"Level"=6, "Class Only"=FALSE, "Identifier"="RSSCOPE_ATTR_ADVANCED_JITTER_RESULTS_COMPONENT_STATISTICS_MIN_PEAK_TO_PEAK", "Descriptive Name"="Advanced Jitter Results Component Statistics Min Peak To Peak", "Data Type"=1, "Command"="ADVJ{AdvJitterMeas}:RES:COMP{AdvJitterComponent}:STAT:MINP?", "Access"=0, "Range Table"="", "Read Callback"="", "Write Callback"="", "Supported Models"="", "Instrument Options"="K133|K134", "Flags"=0, "Help"="Returns the absolute minimum value of the specified measurement component.\n\nAvailable Repeated Capabilities:\nAdvJitterMeas: JA1, JA2\r\nAdvJitterComponent: f_symb, T_symb, EC, TJ_BER, RJ, DDirac, TJ, DJ, DDJ, DCD, PJ, ISI\r\n\nRemote-control command(s):\nADVJitter<m>:RESult:COMPonents<n>:STATistics:MINPeakpeak?"}, {"Level"=6, "Class Only"=FALSE, "Identifier"="RSSCOPE_ATTR_ADVANCED_JITTER_RESULTS_COMPONENT_STATISTICS_MIN_STANDARD_DEVIATION", "Descriptive Name"="Advanced Jitter Results Component Statistics Min Standard Deviation", "Data Type"=1, "Command"="ADVJ{AdvJitterMeas}:RES:COMP{AdvJitterComponent}:STAT:MINS?", "Access"=0, "Range Table"="", "Read Callback"="", "Write Callback"="", "Supported Models"="", "Instrument Options"="K133|K134", "Flags"=0, "Help"="Return the standard deviation of the minimum value of the specified measurement component.\n\nAvailable Repeated Capabilities:\nAdvJitterMeas: JA1, JA2\r\nAdvJitterComponent: f_symb, T_symb, EC, TJ_BER, RJ, DDirac, TJ, DJ, DDJ, DCD, PJ, ISI\r\n\nRemote-control command(s):\nADVJitter<m>:RESult:COMPonents<n>:STATistics[:MINStddev]?"}, {"Level"=5, "Class Only"=TRUE, "Identifier"="", "Descriptive Name"="Scaling", "Data Type"=0, "Command"="", "Access"=0, "Range Table"="", "Read Callback"="", "Write Callback"="", "Supported Models"="", "Instrument Options"="", "Flags"=0, "Help"="This class contains attributes and methods  for configuring the diagrams scales in 
